vi "PPSU Control FGV.vi"(7 "Write/Read":T3=enum."Read", 8 "error in":errorcluster, 11 "PPSU Contol in":T2) -> (0 "error out":errorcluster, 3 "PPSU Control out":T1)   [LabVIEW 2022 SP3]
uses:
  Controls/FGV Read write.ctl
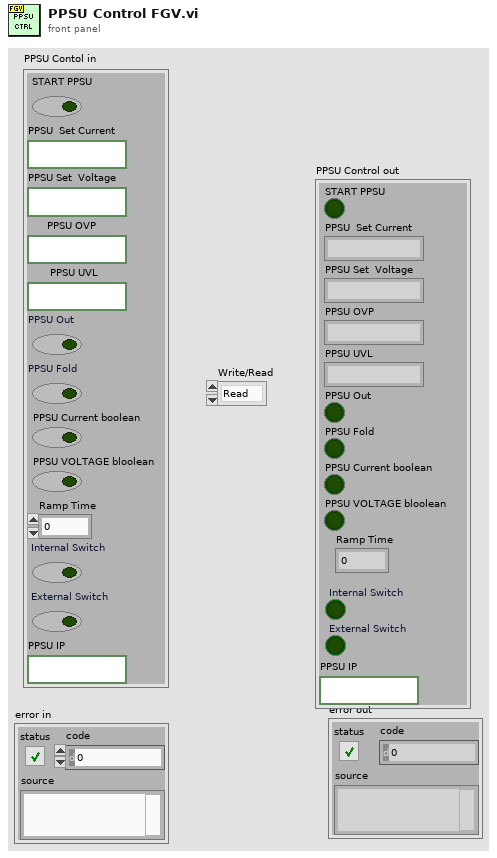
[diagram p1: front panel]
types:
  T1 = cluster{"START PPSU":bool, "PPSU  Set Current":string, "PPSU Set  Voltage":string, "PPSU OVP":string, "PPSU UVL":string, "PPSU Out":bool, "PPSU Fold":bool, "PPSU Current boolean":bool, "PPSU VOLTAGE bloolean":bool, "Ramp Time":dbl, " External Switch ":bool, " Internal Switch ":bool, "PPSU IP":string}
  T2 = cluster{"START PPSU":bool, "PPSU  Set Current":string, "PPSU Set  Voltage":string, "PPSU OVP":string, "PPSU UVL":string, "PPSU Out":bool, "PPSU Fold":bool, "PPSU Current boolean":bool, "PPSU VOLTAGE bloolean":bool, "Ramp Time":dbl, " Internal Switch ":bool, " External Switch ":bool, "PPSU IP":string}
  T3 = typedef "FGV Read write.ctl" = enum16{"Write", "Read"}
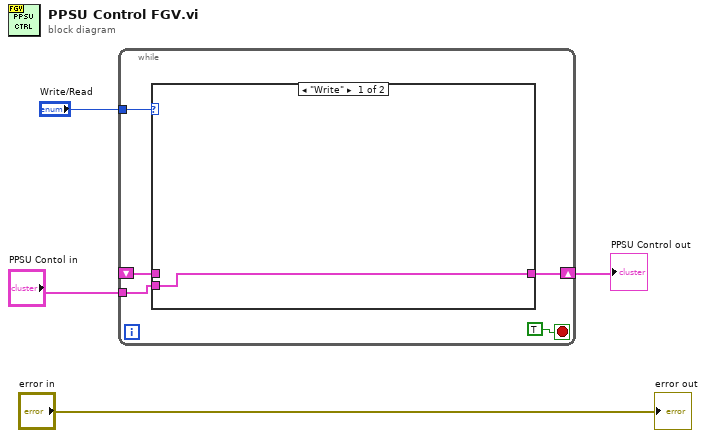
[diagram p0: block diagram]
diagram:
  n1 = while {
    tunnel: "Write/Read" -> [w8]
    shift-right: [w7] -> w1
    shift-left: _ -> [w6]
    tunnel: "PPSU Contol in" -> [w5]
    stop <- TRUE stop-if-true
    n2 = case shown="\"Write\"" w8 {
      tunnel: [w10 w11] -> w7
      tunnel: w6 -> [_ w11]
      tunnel: w5 -> [w10 _]
      frame "Write" {
      }
      frame "Read" {
      }
    }
  }
  "PPSU Control out" <- w1
  "error out" <- "error in"
